vi "Mapping Main.vi"() -> ()   [LabVIEW 2014]
uses:
  C:/Robotic Systems/Products/AgFalcon/Software/Ground Station/Data/Mapping DLL/GMap.NET.Core.dll
  Data/Mapping DLL/GMap.NET.Core.dll
  System.Windows.Forms
  System.Drawing
  C:/Robotic Systems/Products/AgFalcon/Software/Ground Station/Data/Mapping DLL/GMap.NET.WindowsForms.dll
  Data/Mapping DLL/GMap.NET.WindowsForms.dll
panel:
  out "Lng":dbl
  out "Lat":dbl
  in  "Bearing 2":sgl
  out "Imported Map Location":string
  in  "Import Map":path
  out "Bearing":sgl
  out "CacheLocation":string
  out "Height":i32
  out "Width":i32
  in  "Go to New Location":bool
  in  "New Location":string
  out "Route Distance (Km)":dbl
  in  "Create Route":bool
  in  "Set Home":bool
  in  "Draw Polygon":bool
  in  "Clear Markers":bool
  in  "GMapControl":refnum<k24>(container)
  in  "Map Providers":string(combo)
  in  "stop":bool
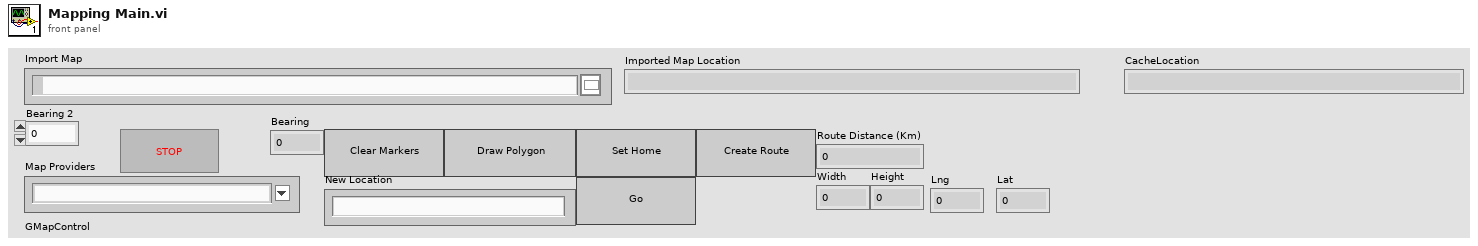
[diagram p1: front panel]
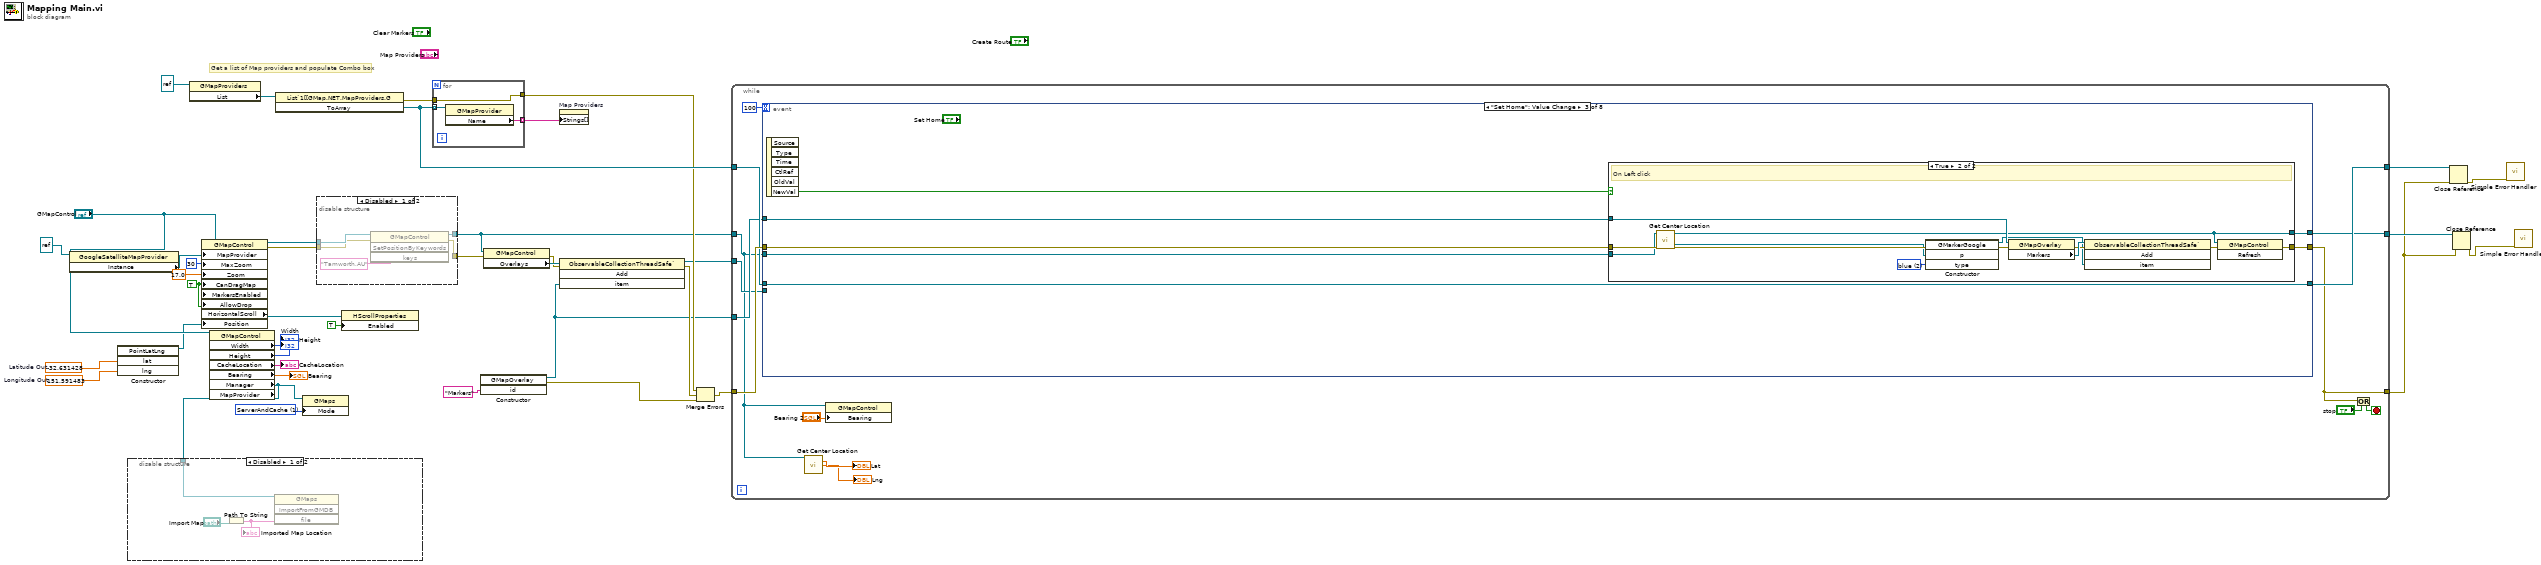
[diagram p0: block diagram]
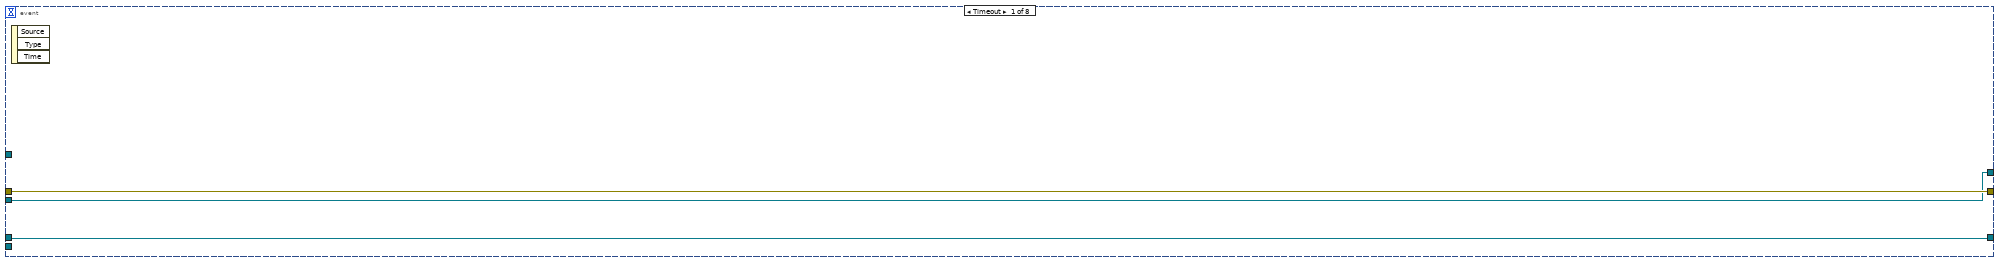
[diagram p4: hidden frame]
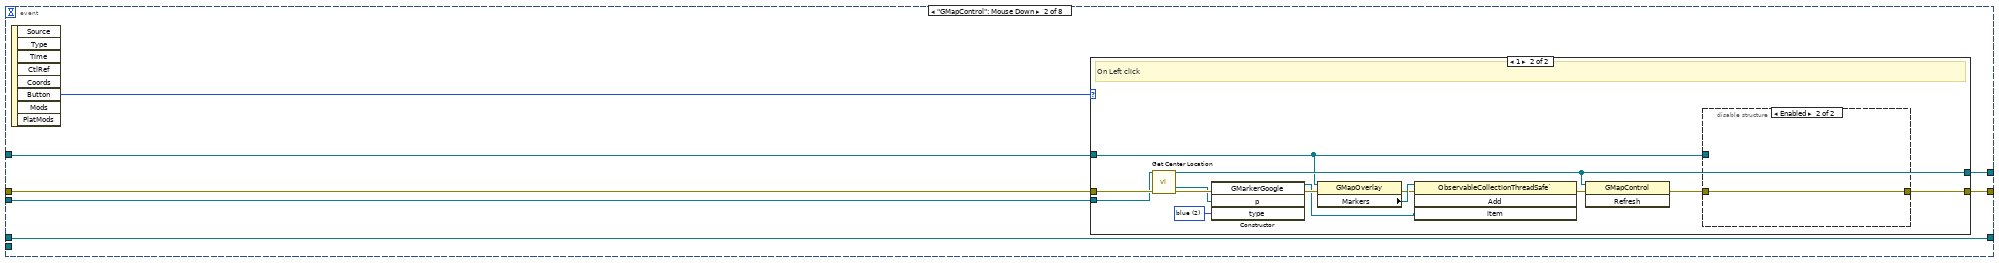
[diagram p5: hidden frame]
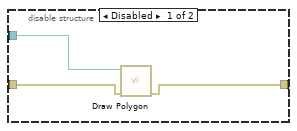
[diagram p7: hidden frame]
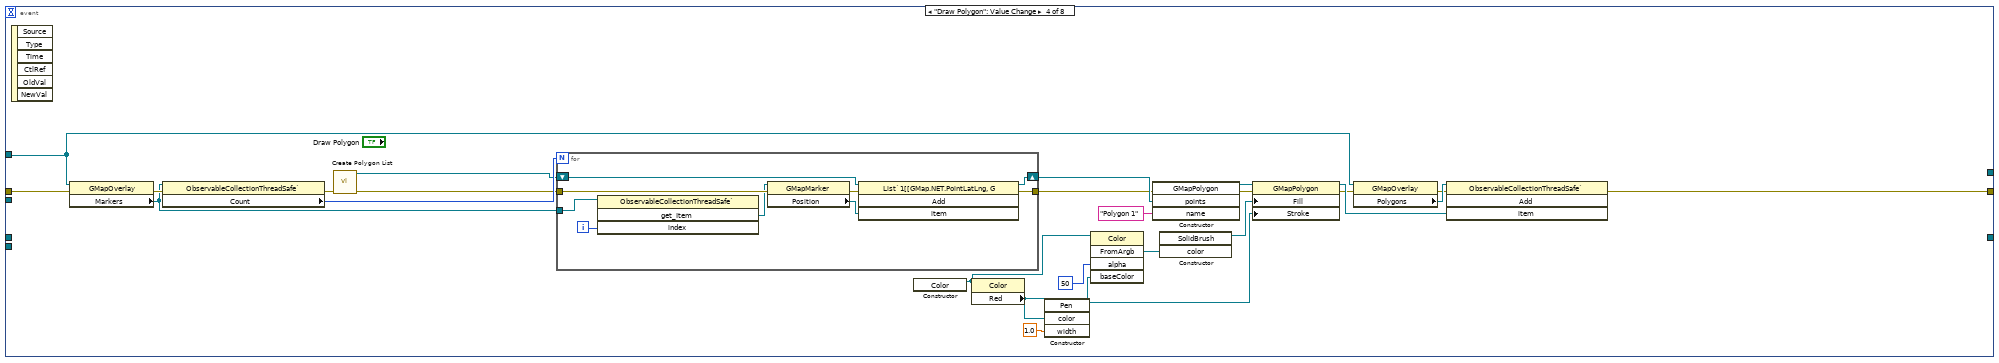
[diagram p9: hidden frame]
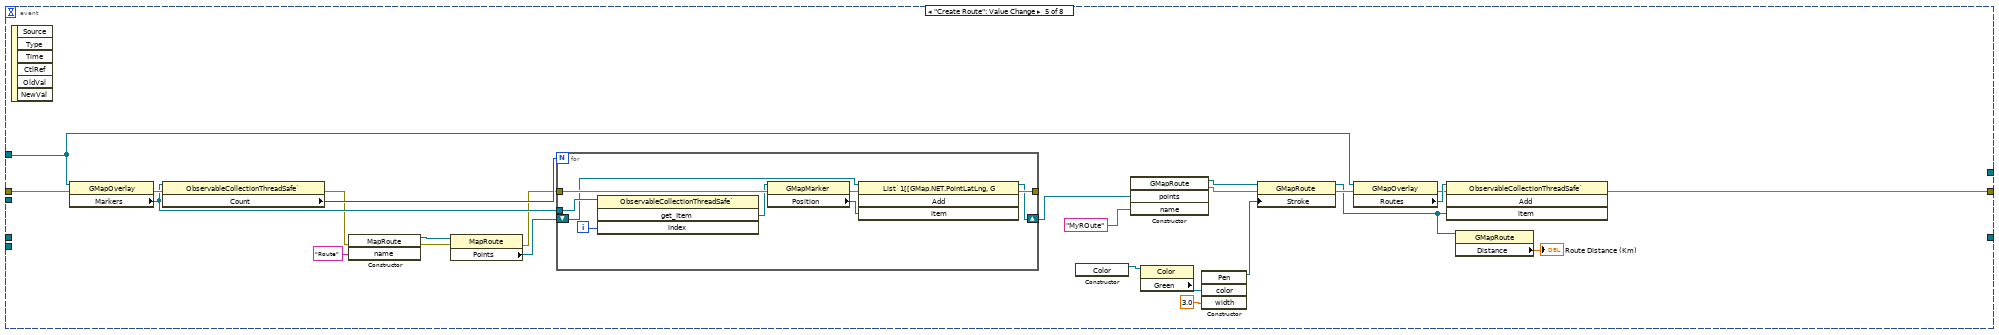
[diagram p10: hidden frame]
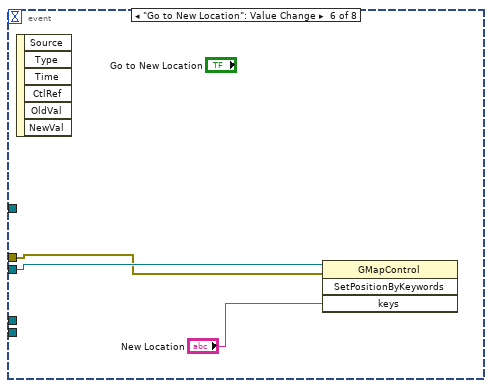
[diagram p11: hidden frame]
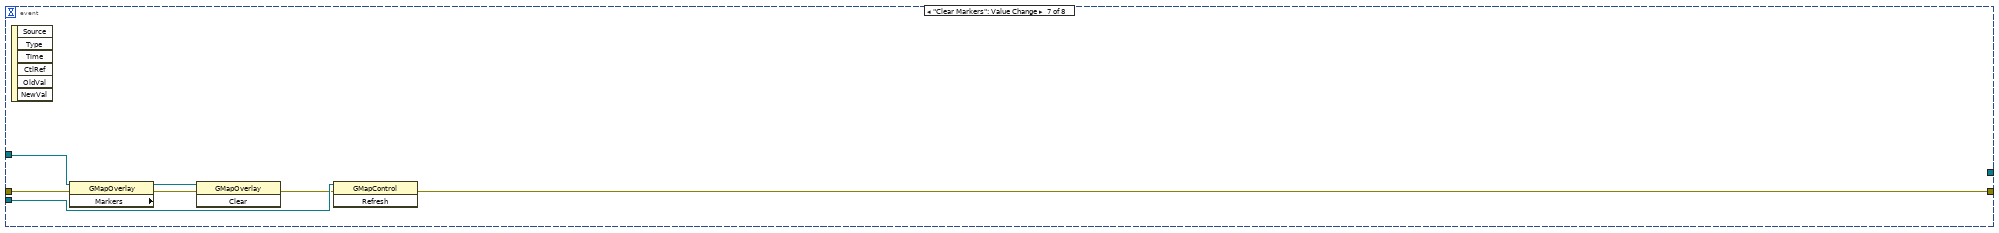
[diagram p12: hidden frame]
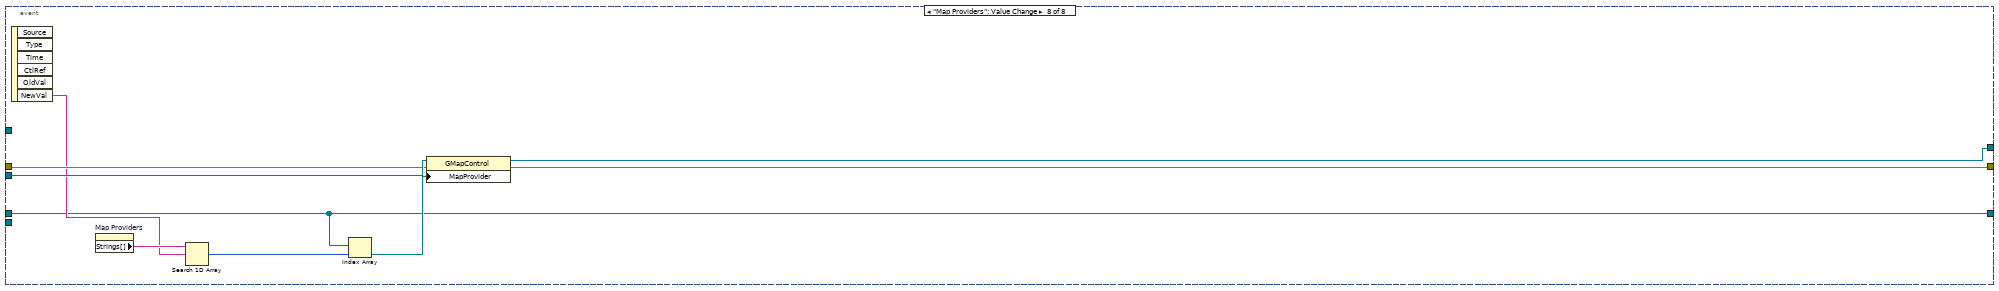
[diagram p13: hidden frame]
diagram:
  w3 = 151.591483  # Longitude Out
  w2 = -32.631428  # Latitude Out
  w5 = 1 items=["ServerOnly", "ServerAndCache", "CacheOnly"] ("Mode")
  w16 = TRUE ("CanDragMap")
  # "Get a list of Map providers and populate Combo box"
  n1 = property class="GoogleSatelliteMapProvider"(reference=refnum<k24> refnum) -> ("Instance"=w33:refnum<k24>)  [unwired: 1 in, 2 out]
  n2 = constructor class="PointLatLng"("lat"=w2, "lng"=w3) -> (reference out=w1:refnum<k24>)  [unwired: 3 in, 4 out]
  n3 = property class="GMapProviders"(reference=refnum<k24> refnum) -> ("List"=w40:refnum<k24>)  [unwired: 1 in, 2 out]
  n4 = property class="GMapControl"(reference="GMapControl", "MapProvider"=w33, "MaxZoom"=30, "Zoom"=17.0, "CanDragMap"=w16, "MarkersEnabled"=w16, "AllowDrop"=w16, "Position"=w1) -> (reference out=w31:refnum<k24>, error out=w30:errorcluster, "HorizontalScroll"=w15:refnum<k24>)  [unwired: 1 in]
  n5 = property class="GMapControl" props=["Width", "Height", "CacheLocation", "Bearing", "Manager", "MapProvider"](reference="GMapControl") -> ("Width"=→"Width":i32, "Height"=→"Height":i32, "CacheLocation"=→"CacheLocation":string, "Bearing"=→"Bearing":sgl, "Manager"=w4:refnum<k24>)  [unwired: 1 in, 3 out]
  n6 = disable-structure shown="Disabled" {
    disable-tunnel: w4 -> [w43 _]
    frame Disabled {
      n7 = Path To String(path="Import Map") -> (string=w42:string)
      "Imported Map Location" <- w42
      n8 = invoke class="GMaps" method="ImportFromGMDB"(reference=w43, "file"=w42) -> ()  [unwired: 2 in, 4 out]
    }
    frame Enabled {
    }
  }
  n9 = invoke class="List`1[[GMap.NET.MapProviders.G" method="ToArray"(reference=w40) -> (error out=w38:errorcluster, "ToArray"=w37:refnum<k24>[])  [unwired: 2 in, 1 out]
  n10 = property class="GMaps"(reference=w4, "Mode"=w5) -> ()  [unwired: 1 in, 2 out]
  n11 = disable-structure shown="Disabled" {
    disable-tunnel: w31 -> [w48 w49]
    disable-tunnel: w30 -> [w47 w50]
    disable-tunnel: [w45 w50] -> w22
    disable-tunnel: [w44 w49] -> w13
    frame Disabled {
      n12 = invoke class="GMapControl" method="SetPositionByKeywords"(reference=w48, error in=w47, "keys"="Tamworth,AU") -> (reference out=w44:refnum<k24>, error out=w45:errorcluster)  [unwired: 1 in, 2 out]
    }
    frame Enabled {
    }
  }
  n13 = property class="HScrollProperties"(reference=w15, "Enabled"=TRUE) -> ()  [unwired: 1 in, 2 out]
  n14 = for {
    tunnel: w37 -> [w53] mode=indexing
    tunnel: [w52] -> w39 mode=indexing
    tunnel: [w51] -> w36
    tunnel: w38 -> [w51]
    n15 = property class="GMapProvider"(reference=w53) -> ("Name"=w52:string)  [unwired: 1 in, 2 out]
  }
  n16 = constructor class="GMapOverlay"("id"="Markers") -> (reference out=w17:refnum<k24>, error out=w18:errorcluster)  [unwired: 3 in, 2 out]
  n17 = property class="GMapControl"(reference=w13, error in=w22) -> (error out=w21:errorcluster, "Overlays"=w23:refnum<k24>)  [unwired: 1 out]
  n18 = property on="Map Providers" class="CmbBox"("Strings[]"=w39) -> ()  [unwired: 2 in, 2 out]
  n19 = invoke class="ObservableCollectionThreadSafe`" method="Add"(reference=w23, error in=w21, "item"=w17) -> (reference out=w12:refnum<k24>, error out=w20:errorcluster)  [unwired: 1 in, 2 out]
  n20 = Merge Errors(w36, w20, w18) -> (w29:errorcluster)
  n21 = while {
    tunnel: w37 -> [w65]
    tunnel: w13 -> [w56]
    tunnel: w29 -> [w66]
    tunnel: [w60] -> w26
    tunnel: [w64] -> w28
    tunnel: [w63] -> w27
    tunnel: w17 -> [w59]
    tunnel: w12 -> [w58]
    stop <- w62 stop-if-true
    n22 = event shown="[2] \"Set Home\": Value Change" {
      selector: _ -> [_ _ _ _ _ _ _ _]
      dyn-events: _ -> [_ _ _ _ _ _ _ _]
      timeout: 100 -> [_ _ _ _ _ _ _ _]
      tunnel: w66 -> [w70 w72 w99 w136 w178 w189 w196 w202]
      tunnel: [w70 w76 w103 w121 w167 _ w191 w200] -> w60
      tunnel: w56 -> [w68 w75 w102 _ _ w190 w193 w203]
      tunnel: w65 -> [w69 w77 w104 _ _ _ _ w198]
      tunnel: [w69 w77 w104 _ _ _ _ w198] -> w64
      tunnel: [w68 w74 w101 _ _ _ _ w199] -> w63
      tunnel: w59 -> [_ w73 w100 w120 w166 _ w197 _]
      tunnel: w58 -> [_ _ _ _ _ _ _ _]
      event Timeout {
        n23 = event-data() -> ()  [unwired: 1 in, 3 out]
      }
      event "GMapControl": Mouse Down {
        n24 = event-data() -> ("Button"=w71:u16)  [unwired: 1 in, 7 out]
        n25 = case shown="1" w71 {
          tunnel: [w78 w81] -> w76
          tunnel: w75 -> [w79 w85]
          tunnel: [w79 w84] -> w74
          tunnel: w73 -> [_ w80]
          tunnel: w72 -> [w78 w88]
          frame 0, Default {
          }
          frame 1 {
            w83 = 2 items=["none", "arrow", "blue", "blue_small", "blue_dot", "blue_pushpin", "brown_small", "gray_small", "green", "green_small", "green_dot", "green_pushpin", "green_big_go", "yellow", "yellow_small", "yellow_dot", "yellow_big_pause", "yellow_pushpin", "lightblue", "lightblue_dot", "lightblue_pushpin", "orange", "orange_small", "orange_dot", "pink", "pink_dot", "pink_pushpin", "purple", "purple_small", "purple_dot", "purple_pushpin", "red", "red_small", "red_dot", "red_pushpin", "red_big_stop", "black_small", "white_small"] ("type")
            # "On Left click"
            n26 = call "Get Center Location.vi"("GMap Control Ref"=w85, "error in (no error)"=w88) -> ("GMap Control Ref Out"=w84:refnum<k24>, "LocationMiddle"=w86:refnum<k24>, "error out"=w87:errorcluster)  [unwired: 9 in, 2 out]
            n27 = constructor class="GMarkerGoogle"(error in=w87, "p"=w86, "type"=w83) -> (reference out=w91:refnum<k24>, error out=w93:errorcluster)  [unwired: 2 in, 3 out]
            n28 = property class="GMapOverlay"(reference=w80, error in=w93) -> (error out=w89:errorcluster, "Markers"=w90:refnum<k24>)  [unwired: 1 out]
            n29 = invoke class="ObservableCollectionThreadSafe`" method="Add"(reference=w90, error in=w89, "item"=w91) -> (error out=w92:errorcluster)  [unwired: 1 in, 3 out]
            n30 = invoke class="GMapControl" method="Refresh"(reference=w84, error in=w92) -> (error out=w82:errorcluster)  [unwired: 1 in, 2 out]
            n31 = disable-structure shown="Enabled" {
              disable-tunnel: w82 -> [w96 w97]
              disable-tunnel: [w95 w97] -> w81
              disable-tunnel: w80 -> [w94 _]
              frame Disabled {
                n32 = call "Draw Polygon.vi"("error in (no error)"=w96, 11:w94) -> ("error out"=w95:errorcluster)  [unwired: 9 in]
              }
              frame Enabled {
              }
            }
          }
        }
      }
      event "Set Home": Value Change {
        n33 = event-data() -> ("NewVal"=w98:bool)  [unwired: 1 in, 5 out]
        n34 = case shown="True" w98 {
          tunnel: [w105 w118] -> w103
          tunnel: w102 -> [w106 w110]
          tunnel: [w106 w109] -> w101
          tunnel: w100 -> [_ w114]
          tunnel: w99 -> [w105 w113]
          frame False {
          }
          frame True {
            w107 = 2 items=["none", "arrow", "blue", "blue_small", "blue_dot", "blue_pushpin", "brown_small", "gray_small", "green", "green_small", "green_dot", "green_pushpin", "green_big_go", "yellow", "yellow_small", "yellow_dot", "yellow_big_pause", "yellow_pushpin", "lightblue", "lightblue_dot", "lightblue_pushpin", "orange", "orange_small", "orange_dot", "pink", "pink_dot", "pink_pushpin", "purple", "purple_small", "purple_dot", "purple_pushpin", "red", "red_small", "red_dot", "red_pushpin", "red_big_stop", "black_small", "white_small"] ("type")
            # "On Left click"
            n35 = call "Get Center Location.vi"("GMap Control Ref"=w110, "error in (no error)"=w113) -> ("GMap Control Ref Out"=w109:refnum<k24>, "LocationMiddle"=w111:refnum<k24>, "error out"=w112:errorcluster)  [unwired: 9 in, 2 out]
            n36 = constructor class="GMarkerGoogle"(error in=w112, "p"=w111, "type"=w107) -> (reference out=w108:refnum<k24>, error out=w119:errorcluster)  [unwired: 2 in, 3 out]
            n37 = property class="GMapOverlay"(reference=w114, error in=w119) -> (error out=w115:errorcluster, "Markers"=w116:refnum<k24>)  [unwired: 1 out]
            n38 = invoke class="ObservableCollectionThreadSafe`" method="Add"(reference=w116, error in=w115, "item"=w108) -> (error out=w117:errorcluster)  [unwired: 1 in, 3 out]
            n39 = invoke class="GMapControl" method="Refresh"(reference=w109, error in=w117) -> (error out=w118:errorcluster)  [unwired: 1 in, 2 out]
          }
        }
      }
      event "Draw Polygon": Value Change {
        n40 = event-data() -> ()  [unwired: 1 in, 6 out]
        n41 = property class="GMapOverlay"(reference=w120, error in=w136) -> (error out=w135:errorcluster, "Markers"=w133:refnum<k24>)  [unwired: 1 out]
        n42 = property class="ObservableCollectionThreadSafe`"(reference=w133, error in=w135) -> (error out=w124:errorcluster, "Count"=w134:i32)  [unwired: 1 out]
        n43 = call "Create Polygon List.vi"("error in (no error)"=w124) -> ("error out"=w123:errorcluster, "specific class reference"=w125:refnum<k24>)  [unwired: 9 in]
        n44 = for {
          N: w134 -> [_]
          tunnel: w123 -> [w150]
          shift-right: [w151] -> w143
          shift-left: w125 -> [w153]
          tunnel: [w148] -> w142
          tunnel: w133 -> [w147]
          i -> [w146]
          n45 = invoke class="ObservableCollectionThreadSafe`" method="get_Item"(reference=w147, "index"=w146) -> ("get_Item"=w145:refnum<k24>)  [unwired: 2 in, 3 out]
          n46 = property class="GMapMarker"(reference=w145, error in=w150) -> (error out=w149:errorcluster, "Position"=w152:refnum<k24>)  [unwired: 1 out]
          n47 = invoke class="List`1[[GMap.NET.PointLatLng, G" method="Add"(reference=w153, error in=w149, "item"=w152) -> (reference out=w151:refnum<k24>, error out=w148:errorcluster)  [unwired: 1 in, 2 out]
        }
        n48 = constructor class="Color"() -> (reference out=w128:refnum<k24>)  [unwired: 3 in, 2 out]
        n49 = property class="Color"(reference=w128) -> ("Red"=w132:refnum<k24>)  [unwired: 1 in, 2 out]
        n50 = constructor class="Pen"("color"=w132, "width"=sgl 1.0 ("Width")) -> (reference out=w130:refnum<k24>)  [unwired: 3 in, 4 out]
        n51 = invoke class="Color" method="FromArgb"(reference=w128, "alpha"=50, "baseColor"=w132) -> ("FromArgb"=w129:refnum<k24>)  [unwired: 2 in, 4 out]
        n52 = constructor class="GMapPolygon"(error in=w142, "points"=w143, "name"="Polygon 1") -> (reference out=w141:refnum<k24>, error out=w140:errorcluster)  [unwired: 2 in, 3 out]
        n53 = constructor class="SolidBrush"("color"=w129) -> (reference out=w139:refnum<k24>)  [unwired: 3 in, 3 out]
        n54 = property class="GMapPolygon"(reference=w141, error in=w140, "Fill"=w139, "Stroke"=w130) -> (reference out=w137:refnum<k24>, error out=w122:errorcluster)
        n55 = property class="GMapOverlay"(reference=w120, error in=w122) -> (error out=w126:errorcluster, "Polygons"=w127:refnum<k24>)  [unwired: 1 out]
        n56 = invoke class="ObservableCollectionThreadSafe`" method="Add"(reference=w127, error in=w126, "item"=w137) -> (error out=w121:errorcluster)  [unwired: 1 in, 3 out]
      }
      event "Create Route": Value Change {
        n57 = event-data() -> ()  [unwired: 1 in, 6 out]
        n58 = property class="GMapOverlay"(reference=w166, error in=w178) -> (error out=w177:errorcluster, "Markers"=w175:refnum<k24>)  [unwired: 1 out]
        n59 = property class="ObservableCollectionThreadSafe`"(reference=w175, error in=w177) -> (error out=w163:errorcluster, "Count"=w176:i32)  [unwired: 1 out]
        n60 = constructor class="MapRoute"(error in=w163, "name"="Route") -> (reference out=w164:refnum<k24>, error out=w162:errorcluster)  [unwired: 2 in, 2 out]
        n61 = property class="MapRoute"(reference=w164, error in=w162) -> (error out=w161:errorcluster, "Points"=w160:refnum<k24>)  [unwired: 1 out]
        n62 = for {
          N: w176 -> [_]
          tunnel: w161 -> [w186]
          tunnel: [w184] -> _
          tunnel: w175 -> [w183]
          shift-right: [w179] -> w159
          shift-left: w160 -> [w180]
          i -> [w182]
          n63 = invoke class="ObservableCollectionThreadSafe`" method="get_Item"(reference=w183, "index"=w182) -> ("get_Item"=w181:refnum<k24>)  [unwired: 2 in, 3 out]
          n64 = property class="GMapMarker"(reference=w181, error in=w186) -> (error out=w185:errorcluster, "Position"=w187:refnum<k24>)  [unwired: 1 out]
          n65 = invoke class="List`1[[GMap.NET.PointLatLng, G" method="Add"(reference=w180, error in=w185, "item"=w187) -> (reference out=w179:refnum<k24>, error out=w184:errorcluster)  [unwired: 1 in, 2 out]
        }
        n66 = constructor class="Color"() -> (reference out=w171:refnum<k24>)  [unwired: 3 in, 2 out]
        n67 = constructor class="GMapRoute"("points"=w159, "name"="MyROute") -> (reference out=w157:refnum<k24>, error out=w156:errorcluster)  [unwired: 3 in, 3 out]
        n68 = property class="Color"(reference=w171) -> ("Green"=w174:refnum<k24>)  [unwired: 1 in, 2 out]
        n69 = constructor class="Pen"("color"=w174, "width"=sgl 3.0 ("Width")) -> (reference out=w172:refnum<k24>)  [unwired: 3 in, 4 out]
        n70 = property class="GMapRoute"(reference=w157, error in=w156, "Stroke"=w172) -> (reference out=w155:refnum<k24>, error out=w168:errorcluster)
        n71 = property class="GMapOverlay"(reference=w166, error in=w168) -> (error out=w169:errorcluster, "Routes"=w170:refnum<k24>)  [unwired: 1 out]
        n72 = invoke class="ObservableCollectionThreadSafe`" method="Add"(reference=w170, error in=w169, "item"=w155) -> (error out=w167:errorcluster)  [unwired: 1 in, 3 out]
        n73 = property class="GMapRoute"(reference=w155) -> ("Distance"=→"Route Distance (Km)":dbl)  [unwired: 1 in, 2 out]
      }
      event "Go to New Location": Value Change {
        n74 = event-data() -> ()  [unwired: 1 in, 6 out]
        n75 = invoke class="GMapControl" method="SetPositionByKeywords"(reference=w190, error in=w189, "keys"="New Location") -> ()  [unwired: 1 in, 4 out]
      }
      event "Clear Markers": Value Change {
        n76 = event-data() -> ()  [unwired: 1 in, 6 out]
        n77 = property class="GMapOverlay" props=["Markers"](reference=w197, error in=w196) -> (reference out=w195:refnum<k24>, error out=w194:errorcluster)  [unwired: 1 out]
        n78 = invoke class="GMapOverlay" method="Clear"(reference=w195, error in=w194) -> (error out=w192:errorcluster)  [unwired: 1 in, 2 out]
        n79 = invoke class="GMapControl" method="Refresh"(reference=w193, error in=w192) -> (error out=w191:errorcluster)  [unwired: 1 in, 2 out]
      }
      event "Map Providers": Value Change {
        n80 = event-data() -> ("NewVal"=w201:string)  [unwired: 1 in, 5 out]
        n81 = property on="Map Providers" class="CmbBox"() -> ("Strings[]"=w206:string[])  [unwired: 2 in, 2 out]
        n82 = Search 1D Array(1D array=w206, element=w201) -> (index of element=w204:i32)  [unwired: 1 in]
        n83 = Index Array(array=w198, index=w204) -> (element=w205:refnum<k24>)
        n84 = property class="GMapControl"(reference=w203, error in=w202, "MapProvider"=w205) -> (reference out=w199:refnum<k24>, error out=w200:errorcluster)
      }
    }
    n85 = call "Get Center Location.vi"("GMap Control Ref"=w56) -> ("Lat"=→"Lat":dbl, "Lng"=→"Lng":dbl)  [unwired: 10 in, 3 out]
    n86 = property class="GMapControl"(reference=w56, "Bearing"="Bearing 2") -> ()  [unwired: 1 in, 2 out]
    n87 = Or(x=w60, y="stop") -> (x .or. y?=w62:bool)
  }
  n88 = Close Reference(reference=w28, error in (no error)=w26) -> (error out=w25:errorcluster)
  n89 = Close Reference(reference=w27, error in (no error)=w26) -> (error out=w24:errorcluster)
  n90 = call <vilib>:"Simple Error Handler.vi"("error in (no error)"=w25) -> ()  [unwired: 4 in, 5 out]
  n91 = call <vilib>:"Simple Error Handler.vi"("error in (no error)"=w24) -> ()  [unwired: 4 in, 5 out]
